vi "Get Row Stride.vi"(11 "Image":T1) -> (2 "Padded Width":i32, 3 "Row Stride":i32)   [LabVIEW 2020, in "G-Image.lvlib"]
doc: "Get the number of bytes which make up a row in the image data 1D array, and the width of the image including padding. Note that the stride can be longer than (image width * channels) due to padding."
uses:
  G-Image.lvlib
  <vilib>/picture/picture.llb/imagedata.ctl
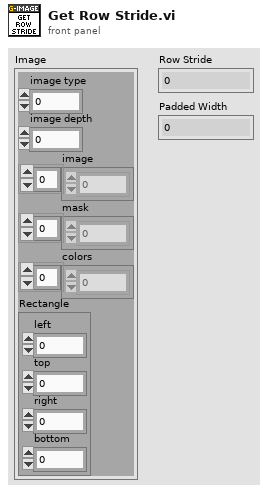
[diagram p1: front panel]
types:
  T1 = typedef "imagedata.ctl" = cluster{"image type":i32, "image depth":i32, "image":u8[], "mask":u8[], "colors":u32[], "Rectangle":cluster{"left":i16, "top":i16, "right":i16, "bottom":i16}}
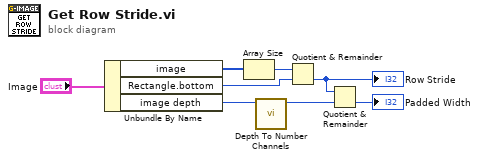
[diagram p0: block diagram]
diagram:
  n1 = Unbundle By Name("Image") -> ("image"=w7:u8[], "Rectangle.bottom"=w5:i16, "image depth"=w3:i32)
  n2 = Array Size(array=w7) -> (size(s)=w6:i32)
  n3 = call "Depth To Number Channels.vi"("Depth"=w3) -> ("Channels"=w2:i32)  [unwired: 10 in]
  n4 = Quotient & Remainder(x=w6, y=w5) -> (floor(x/y)=w4:i32)  [unwired: 1 out]
  "Row Stride" <- w4
  n5 = Quotient & Remainder(x=w4, y=w2) -> (floor(x/y)=→"Padded Width":i32)  [unwired: 1 out]
